vi "ClusterElementNames.vi"(8 "error in":errorcluster, 11 "input cluster":variant) -> (0 "error out":errorcluster, 2 "DataTypes":T1[](array[typedef]), 3 "Elements Names":string[](array[string]))   [LabVIEW 2013]
uses:
  <vilib>/Utility/VariantDataType/Type.ctl
  <vilib>/Utility/VariantDataType/VariantType.lvlib
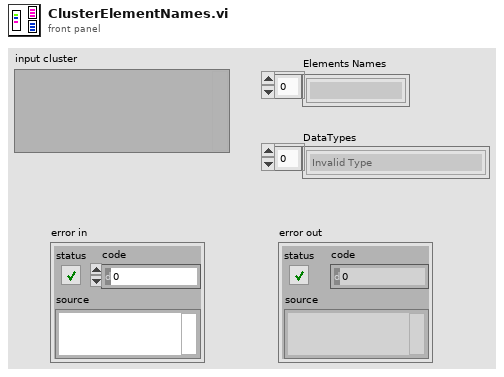
[diagram p1: front panel]
types:
  T1 = typedef "VariantType.lvlib/Type.ctl" = enum8{"Invalid Type", "Void", "I8", "I16", "I32", "I64", "U8", "U16", "U32", "U64", "Single Float", "Double Float", "Extended Float", "Single Complex", "Double Complex", "Extended Complex", "Enum U8", "Enum U16", "Enum U32", "Enum U64", "Single Float With Unit", "Double Float With Unit", "Extended Float With Unit", "Single Complex with Unit", "Double Complex with Unit", "Extended Complex with Unit", "Boolean", "String", "Path", "Picture", "Tag", "Array", "Cluster", "Variant", "LV Variant", "Waveform", "Timestamp", "Digital Waveform", "Digital Data", "ExpressData", "Refnum", "External Data", "VI", "Poly VI", "LabVIEW Class Instance", "Fixed Point"}
  T2 = typedef "tag bus.lvlib/tag descriptor.lvclass/Data Type.ctl" = enum16{"Double", "Single", "I64", "I32", "I16", "I8", "U64", "U32", "U16", "U8", "Boolean", "String", "Array of Double", "Array of Single", "Array of I64", "Array of I32", "Array of I16", "Array of I8", "Array of U64", "Array of U32", "Array of U16", "Array of U8", "Array of Boolean", "Array of String"}
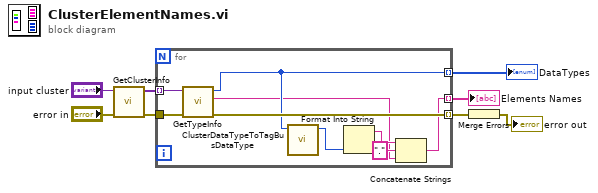
[diagram p0: block diagram]
diagram:
  n1 = call <vilib>:"GetClusterInfo.vi"("error in (no error)"="error in", "Variant"="input cluster") -> ("error out"=w4:errorcluster, "Cluster Elements"=w7:variant[])  [unwired: 8 in]
  n2 = for {
    tunnel: w7 -> [w17] mode=indexing
    tunnel: [w14] -> w1 mode=indexing
    tunnel: [w9] -> w6 mode=indexing
    tunnel: w4 -> [w16]
    tunnel: [w15] -> w3 mode=indexing
    n3 = call <vilib>:"GetTypeInfo.vi"("error in (no error)"=w16, "Variant"=w17) -> ("error out"=w15:errorcluster, "Name"=w10:string, "Type Enum"=w14:T1)  [unwired: 5 in, 2 out]
    n4 = call "ClusterDataTypeToTagBusDataType.vi"("Type Enum"=w14) -> ("data type"=w13:T2)  [unwired: 10 in]
    n5 = Format Into String(w13) -> (resulting string=w12:string)  [unwired: 3 in, 1 out]
    n6 = Concatenate Strings(w12, "." ("string"), w10) -> (w9:string)
  }
  "Elements Names" <- w6
  "DataTypes" <- w1
  n7 = Merge Errors(w3) -> (→"error out":errorcluster)
